vi "NT Delete Entry.vi"(8 "error in":errorcluster, 10 "All":bool, 11 "Name":string="Numeric") -> (0 "error out":errorcluster)   [LabVIEW 2017]
doc: "Write the double precision numeric to the named entry."
uses:
  <vilib>/Rock Robotics/Network Tables/Make Table Operation.ctl
  <vilib>/Rock Robotics/Network Tables/Create Actual Table Name.vi
  <vilib>/Rock Robotics/Network Tables/NT Globals.vi
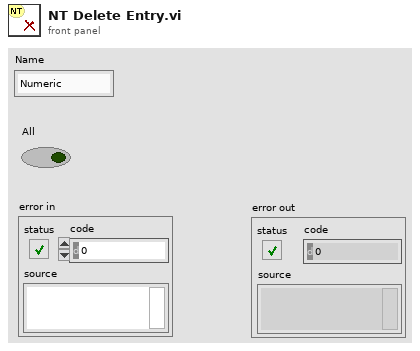
[diagram p1: front panel]
types:
  T1 = typedef "Make Table Operation.ctl" = enum16{"Get or Add Field", "Get Field or Add Temp", "Replace Temp ID", "Get Field ID - No Add", "Get Table Field IDs", "Get Field ID Info", "Move Field to Temp", "Validate", "Remove Field", "Remove All"}
  T2 = enum16{"Update Field", "Read Field", "Assign Field", "Remove All", "Set Persistence", "Clear Persistence"}
  T3 = typedef "Field ID.ctl" = i32
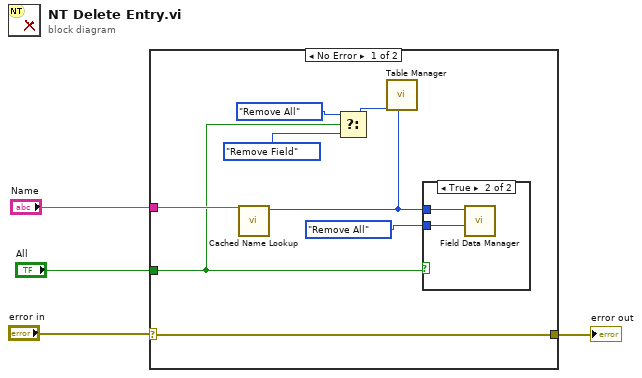
[diagram p0: block diagram]
diagram:
  n1 = case shown="No Error" "error in" {
    selector: "error in" -> [w12 w15]
    tunnel: "All" -> [w6 _]
    tunnel: "Name" -> [w8 _]
    tunnel: [w12 w15] -> w2
    frame No Error {
      n2 = call <vilib>:"Cached Name Lookup.vi"("Name"=w8) -> ("Entry ID"=w7:T3)  [unwired: 8 in, 2 out]
      n3 = Select(t=Make_Table_Operation."Remove All" ("Operation"), s=w6, f=Make_Table_Operation."Remove Field" ("Operation")) -> (s? t:f=w9:T1)
      n4 = call <vilib>:"Table Manager.vi"("Entry ID in"=w7, "Operation"=w9) -> ()  [unwired: 6 in, 4 out]
      n5 = case shown="True" w6 {
        tunnel: T2."Remove All" ("Operation") -> [_ w14]
        tunnel: w7 -> [_ w13]
        frame False {
        }
        frame True {
          n6 = call <vilib>:"Field Data Manager.vi"("Operation"=w14, "Field ID"=w13) -> ()  [unwired: 8 in, 2 out]
        }
      }
    }
    frame Error {
    }
  }
  "error out" <- w2
